vi "Align To Connector Pane Sub.vi"(7 "QD Launch VI Panel?":bool, 8 "error in (no error)":errorcluster, 9 "Changed In":bool, 10 "QD Combo Box Ref":refnum<vi>, 11 "VI in":refnum<vi>) -> (0 "error out":errorcluster, 1 "Changed Out":bool, 3 "VI out":refnum<vi>)   [LabVIEW 2017]
uses:
  Align To Connector Pane Sub VIs/Align To Connector.lvlib
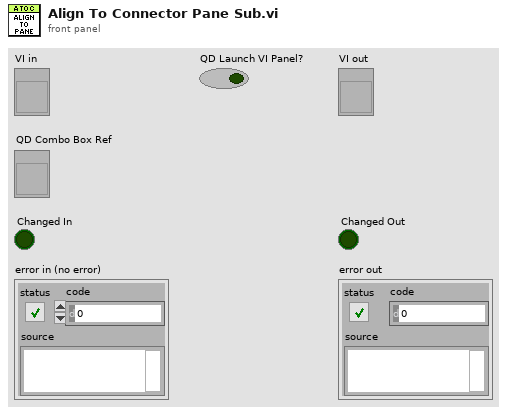
[diagram p1: front panel]
types:
  T1 = typedef "LVPositionTypeDef.ctl" = cluster{"Left":i32, "Top":i32}
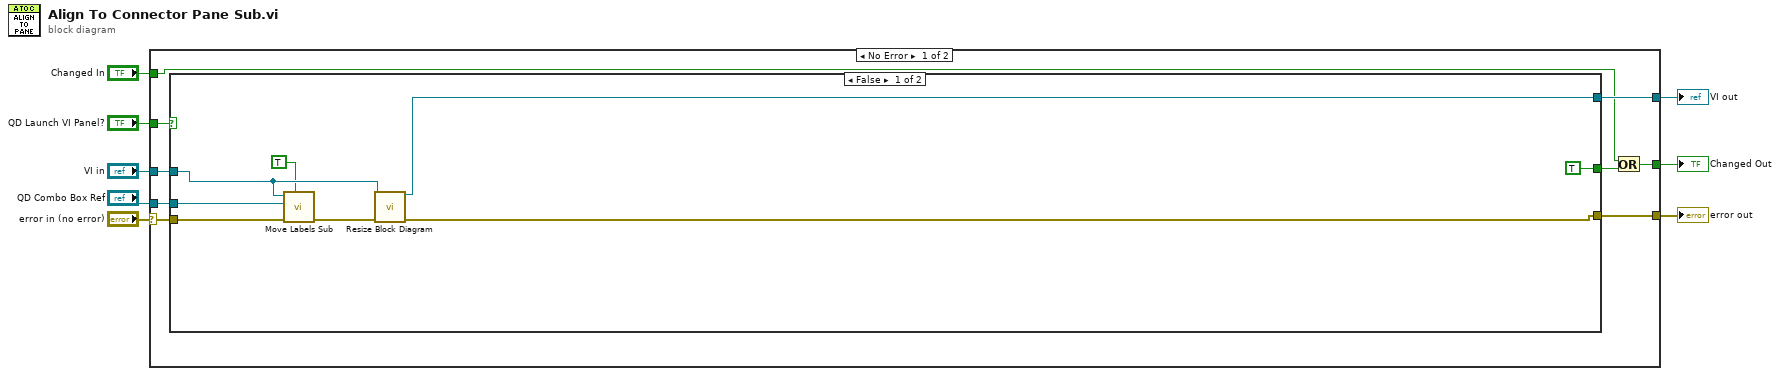
[diagram p0: block diagram]
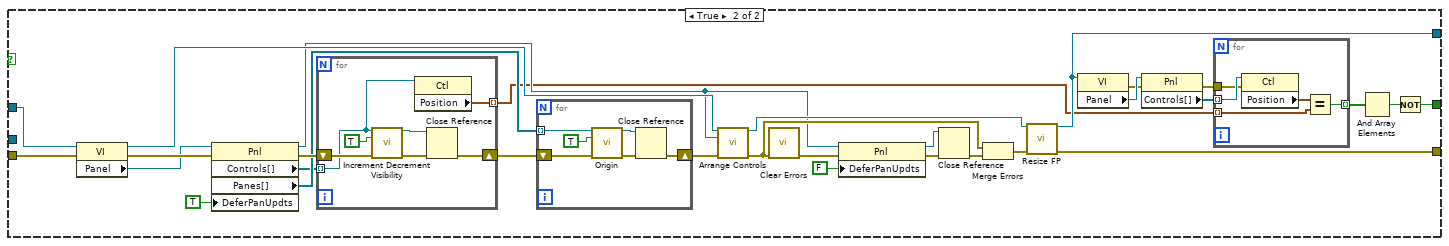
[diagram p2: hidden frame]
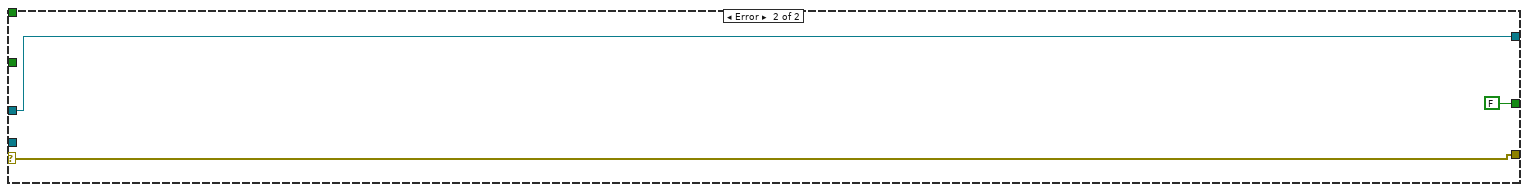
[diagram p3: hidden frame]
diagram:
  n1 = case shown="No Error" "error in (no error)" {
    selector: "error in (no error)" -> [w13 w76]
    tunnel: [w17 w76] -> w8
    tunnel: "QD Launch VI Panel?" -> [w16 _]
    tunnel: [w15 w75] -> w6
    tunnel: "VI in" -> [w14 w75]
    tunnel: [w12 FALSE] -> w3
    tunnel: "Changed In" -> [w11 _]
    tunnel: "QD Combo Box Ref" -> [w9 _]
    frame No Error {
      n2 = case shown="False" w16 {
        tunnel: w13 -> [w22 w36]
        tunnel: w14 -> [w20 w37]
        tunnel: [w24 w34] -> w15
        tunnel: [w25 w42] -> w17
        tunnel: [TRUE w27] -> w10
        tunnel: w9 -> [w18 _]
        frame False {
          n3 = call "Move Labels Sub.vi"("Shift Pressed?"=TRUE, "error in (no error)"=w22, "QD Combo Box Ref"=w18, "QD Launch VI Ref"=w20) -> ("error out"=w21:errorcluster)  [unwired: 6 in, 1 out]
          n4 = call "Resize Block Diagram.vi"("VI in"=w20, "error in"=w21) -> ("VI out"=w24:refnum<vi>, "error out"=w25:errorcluster)  [unwired: 12 in]
        }
        frame True {
          n5 = property class="VI"(reference=w37, error in=w36) -> (reference out=w41:refnum<vi>, error out=w55:errorcluster, "Panel"=w54:refnum<vi>)
          n6 = property class="Pnl"(reference=w54, error in=w55, "DeferPanUpdts"=TRUE ("Defer Panel Updates")) -> (reference out=w40:refnum<vi>, error out=w48:errorcluster, "Controls[]"=w35:refnum<vi>[], "Panes[]"=w46:refnum<vi>[])
          n7 = for {
            tunnel: w35 -> [w62] mode=indexing
            shift-right: [w67] -> w47
            shift-left: w48 -> [w64]
            tunnel: [w61] -> w31 mode=indexing
            n8 = call "Increment Decrement Visibility.vi"("Control in"=w62, "make compliant?"=TRUE, "error in"=w64) -> ("Control out"=w66:refnum<vi>, "error out"=w65:errorcluster)  [unwired: 10 in, 1 out]
            n9 = property class="Ctl"(reference=w62) -> ("Position"=w61:T1)  [unwired: 1 in, 2 out]
            n10 = Close Reference(reference=w66, error in (no error)=w65) -> (error out=w67:errorcluster)
          }
          n11 = for {
            tunnel: w46 -> [w70] mode=indexing
            shift-right: [w73] -> w45
            shift-left: w47 -> [w69]
            n12 = call "Origin.vi"("Pane in"=w70, "make compliant?"=TRUE, "error in"=w69) -> ("Pane out"=w72:refnum<vi>, "error out"=w71:errorcluster)  [unwired: 10 in, 1 out]
            n13 = Close Reference(reference=w72, error in (no error)=w71) -> (error out=w73:errorcluster)
          }
          n14 = call "Arrange Controls.vi"("VI in"=w41, "front panel"=w40, "error in"=w45) -> ("VI out"=w49:refnum<vi>, "error out"=w44:errorcluster)  [unwired: 11 in]
          n15 = call <vilib>:"Clear Errors.vi"("error in (no error)"=w44) -> ("error out"=w43:errorcluster)  [unwired: 5 in, 1 out]
          n16 = property class="Pnl"(reference=w40, error in=w43, "DeferPanUpdts"=FALSE ("Defer Panel Updates")) -> (reference out=w51:refnum<vi>, error out=w52:errorcluster)
          n17 = Close Reference(reference=w51, error in (no error)=w52) -> (error out=w39:errorcluster)
          n18 = Merge Errors(w44, w39) -> (w38:errorcluster)
          n19 = call "Resize FP.vi"("VI in"=w49, "error in"=w38) -> ("VI out"=w34:refnum<vi>, "error out"=w42:errorcluster)  [unwired: 12 in]
          n20 = property class="VI"(reference=w34) -> (error out=w26:errorcluster, "Panel"=w33:refnum<vi>)  [unwired: 1 in, 1 out]
          n21 = property class="Pnl"(reference=w33, error in=w26) -> (error out=w30:errorcluster, "Controls[]"=w32:refnum<vi>[])  [unwired: 1 out]
          n22 = for {
            tunnel: w32 -> [w60] mode=indexing
            tunnel: w31 -> [w57] mode=indexing
            tunnel: w30 -> [w59]
            tunnel: [w56] -> w29 mode=indexing
            n23 = property class="Ctl"(reference=w60, error in=w59) -> ("Position"=w58:T1)  [unwired: 2 out]
            n24 = Equal?(x=w58, y=w57) -> (x = y?=w56:bool)
          }
          n25 = And Array Elements(Boolean array=w29) -> (logical AND=w28:bool)
          n26 = Not(x=w28) -> (.not. x?=w27:bool)
        }
      }
      n27 = Or(x=w11, y=w10) -> (x .or. y?=w12:bool)
    }
    frame Error {
    }
  }
  "error out" <- w8
  "VI out" <- w6
  "Changed Out" <- w3
